vi "rs3 init downsample.vi"(8 "error in (no error)":errorcluster) -> (0 "error out":errorcluster, 1 "error frame queue":u64, 2 "error decimation block":u64, 3 "error start processing":u64, 4 "decimation filter block":u64, 5 "decimation filter queue":u64)   [LabVIEW 2018, in "libRealSense3.lvlib"]
doc: "Initialized processing block & queue for down-sampling the output depth"
uses:
  libRealSense3.lvlib
  realsense2.dll
panel:
  # "RS3 Init DownSample"
  # "(C) Intel Corp.,  AGJ"
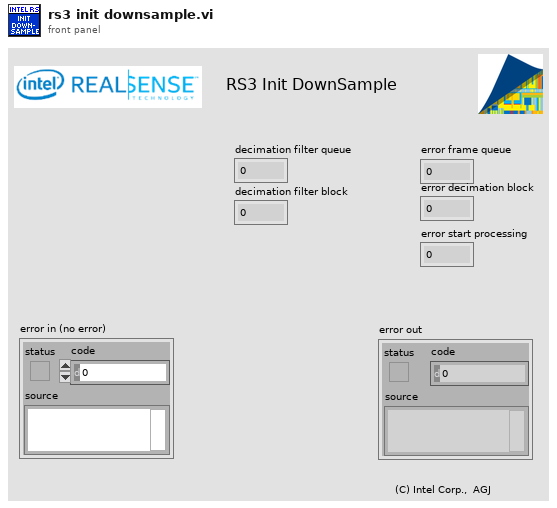
[diagram p1: front panel]
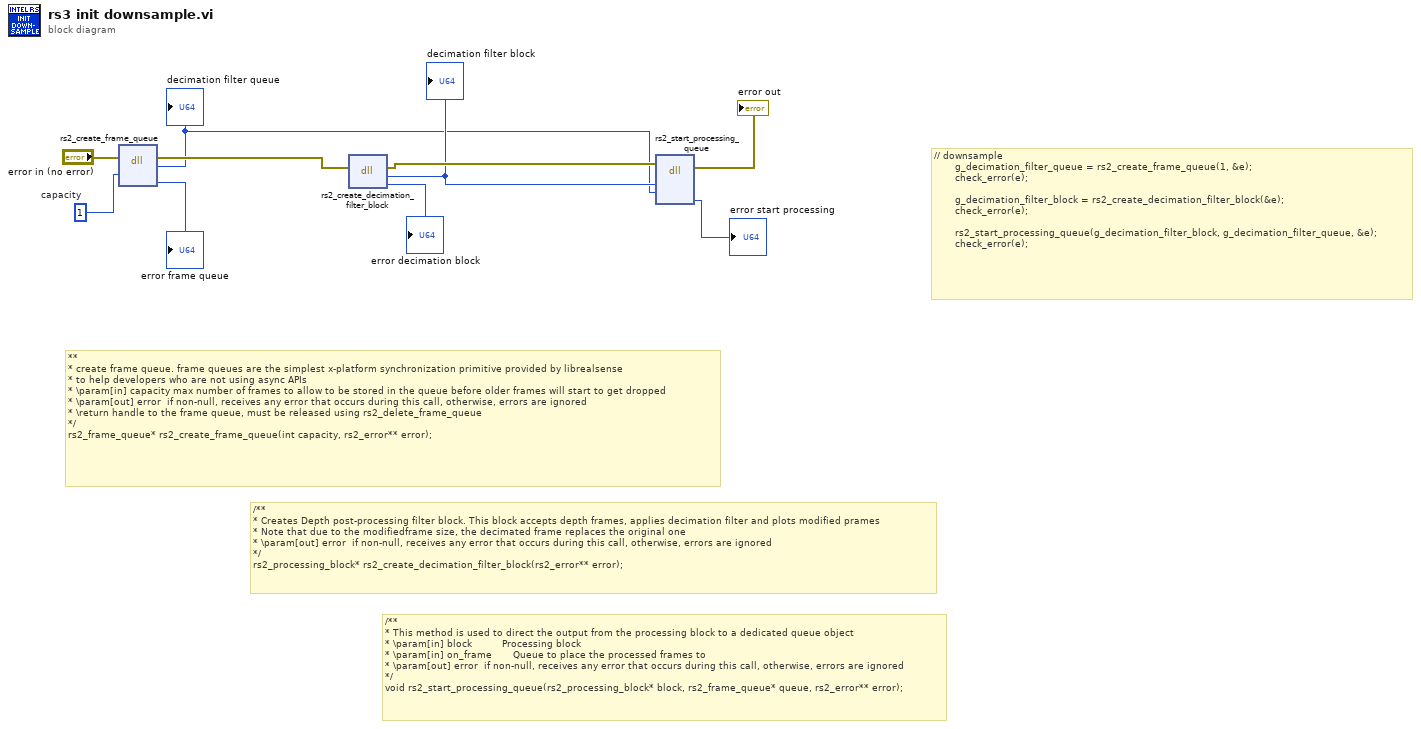
[diagram p0: block diagram]
diagram:
  w9 = 1  # capacity
  # "/**\n* This method is used to direct the output from the processing block to a dedicated queue object\n* \\param[in] block          Processing block\n* \\param[in] on_frame       Queue to place the processed frames to\n* \\param[out] error  if non-null, receives any error that occurs during this call, otherwise, errors are ignored\n*/\nvoid rs2_start_processing_queue(rs2_processing_block* block, rs2_frame_queue* queue, rs2_error** error);"
  # "/**\n* Creates Depth post-processing filter block. This block accepts depth frames, applies decimation filter and plots modified prames\n* Note that due to the modifiedframe size, the decimated frame replaces the original one\n* \\param[out] error  if non-null, receives any error that occurs during this call, otherwise, errors are ignored\n*/\nrs2_processing_block* rs2_create_decimation_filter_block(rs2_error** error);"
  # "**\n* create frame queue. frame queues are the simplest x-platform synchronization primitive provided by librealsense\n* to help developers who are not using async APIs\n* \\param[in] capacity max number of frames to allow to be stored in the queue before older frames will start to get dropped\n* \\param[out] error  if non-null, receives any error that occurs during this call, otherwise, errors are ignored\n* \\return handle to the frame queue, must be released using rs2_delete_frame_queue\n*/\nrs2_frame_queue* rs2_create_frame_queue(int capacity, rs2_error** error);"
  # "// downsample\n       g_decimation_filter_queue = rs2_create_frame_queue(1, &e);\n       check_error(e);\n\n       g_decimation_filter_block = rs2_create_decimation_filter_block(&e);\n       check_error(e);\n\n       rs2_start_processing_queue(g_decimation_filter_block, g_decimation_filter_queue, &e);\n       check_error(e);"
  n1 = dll-call lib="C:/Users/aaron.jencks/Documents/GitHub/emerson_seed_object_detection/LabVIEW/Projects/Paul's Video Viewer/Classes/Realsense Cam/realsense_wrapper_api/realsense2.dll" fn="rs2_create_frame_queue"(error in="error in (no error)", "capacity"=w9) -> (error out=w7:errorcluster, "decimation filter queue"=w2:u64, "error"=→"error frame queue":u64)  [unwired: 4 in, 1 out]
  "decimation filter queue" <- w2
  n2 = dll-call lib="C:/Users/aaron.jencks/Documents/GitHub/emerson_seed_object_detection/LabVIEW/Projects/Paul's Video Viewer/Classes/Realsense Cam/realsense_wrapper_api/realsense2.dll" fn="rs2_create_decimation_filter_block"(error in=w7) -> (error out=w5:errorcluster, "decimation filter block"=w3:u64, "error"=→"error decimation block":u64)  [unwired: 3 in, 1 out]
  "decimation filter block" <- w3
  n3 = dll-call lib="C:/Users/aaron.jencks/Documents/GitHub/emerson_seed_object_detection/LabVIEW/Projects/Paul's Video Viewer/Classes/Realsense Cam/realsense_wrapper_api/realsense2.dll" fn="rs2_start_processing_queue"(error in=w5, "processing block"=w3, "frame queue"=w2) -> (error out=→"error out":errorcluster, "error"=→"error start processing":u64)  [unwired: 6 in, 1 out]
